vi "tip-down-trigger_from_ref.vi"(9 "TOL":sgl, 10 "setpoint":sgl, 11 "I/O Item":fxp<+/-,24,5>) -> (3 "Boolean":bool)   [LabVIEW 2017]
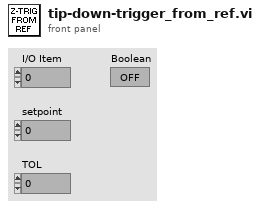
[diagram p1: front panel]
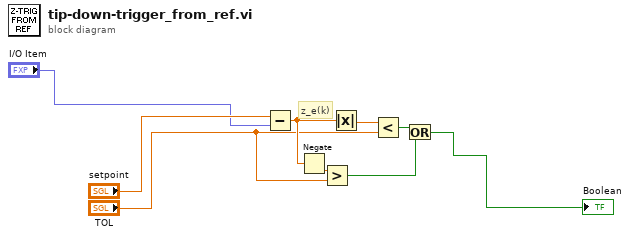
[diagram p0: block diagram]
diagram:
  # "z_e(k)"
  n1 = Subtract(x="setpoint", y="I/O Item") -> (x-y=w9:sgl)
  n2 = Negate(x=w9) -> (-x=w8:sgl)
  n3 = Greater?(x=w8, y="TOL") -> (0:w7:bool)
  n4 = Absolute Value(x=w9) -> (abs(x)=w5:sgl)
  n5 = Less?(x=w5, y="TOL") -> (x < y?=w6:bool)
  n6 = Or(x=w6, y=w7) -> (x .or. y?=→"Boolean":bool)
